vi "FGV - Trigger.vi"(4 "error in":errorcluster, 6 "Function":enum16{"write", "read"}(ring), 7 "Trigger":bool) -> (0 "error out":errorcluster, 3 "Trigger 2":bool)   [LabVIEW 2016]
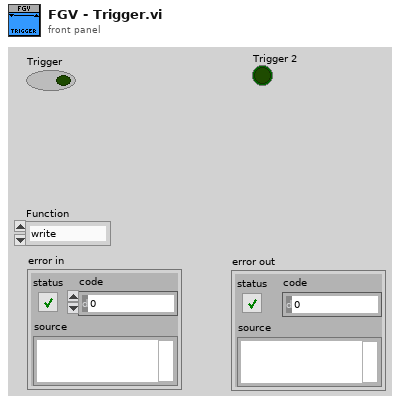
[diagram p1: front panel]
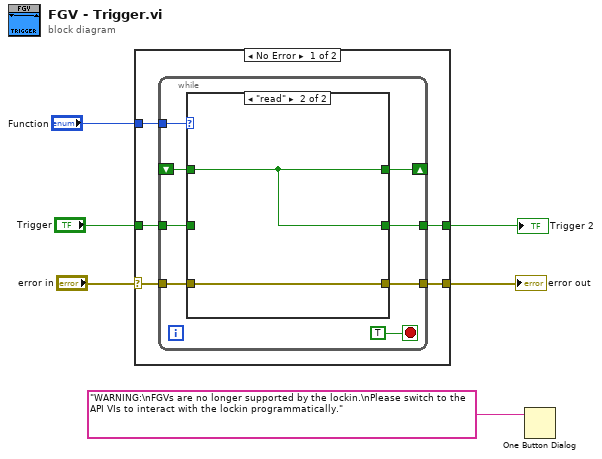
[diagram p0: block diagram]
diagram:
  n1 = case shown="No Error" "error in" {
    selector: "error in" -> [w11 w25]
    tunnel: [w10 w25] -> w5
    tunnel: "Trigger" -> [w9 w24]
    tunnel: [w8 w24] -> w4
    tunnel: "Function" -> [w7 _]
    frame No Error {
      n2 = while {
        shift-right: [w13] -> _
        shift-left: _ -> [w12]
        tunnel: w11 -> [w18]
        tunnel: [w17] -> w10
        tunnel: w9 -> [w16]
        tunnel: [w15] -> w8
        tunnel: w7 -> [w14]
        stop <- TRUE stop-if-true
        n3 = case shown="\"read\"" w14 {
          tunnel: w18 -> [w20 w23]
          tunnel: [w20 w23] -> w17
          tunnel: w16 -> [w21 _]
          tunnel: [w21 w22] -> w15
          tunnel: [w21 w22] -> w13
          tunnel: w12 -> [_ w22]
          frame "write", Default {
          }
          frame "read" {
          }
        }
      }
    }
    frame Error {
    }
  }
  "error out" <- w5
  "Trigger 2" <- w4
  n4 = One Button Dialog(message="WARNING:\nFGVs are no longer supported by the lockin.\nPlease switch to the API VIs to interact with the lockin programmatically.") -> ()  [unwired: 1 in, 1 out]
